vi "IsSetter.vi"(8 "error in (no error)":errorcluster, 10 "Path":path, 11 "ClassReflector in":refnum<class "ClassReflector.lvclass">) -> (0 "error out":errorcluster, 1 "IsSetter?":bool, 3 "ClassReflector out":refnum<class "ClassReflector.lvclass">)   [LabVIEW 2023, in "ClassReflector.lvclass"]
uses:
  ClassReflector.lvclass
  ClassReflector.lvclass/ClassReflector.ctl
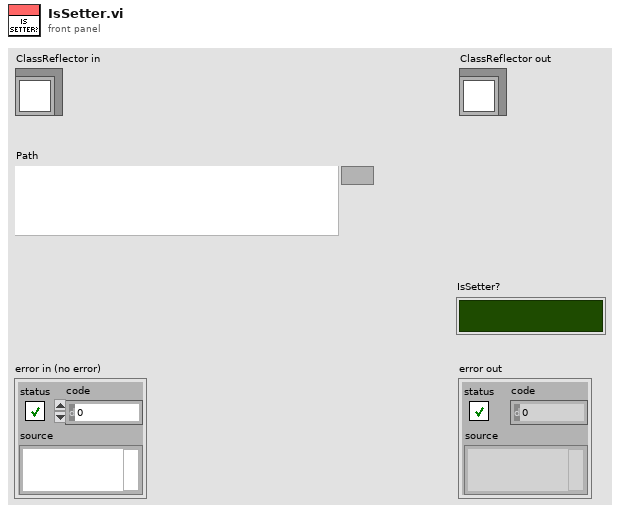
[diagram p1: front panel]
types:
  T1 = enum32{"Bad", "Idle", "Run top level", "Running"}
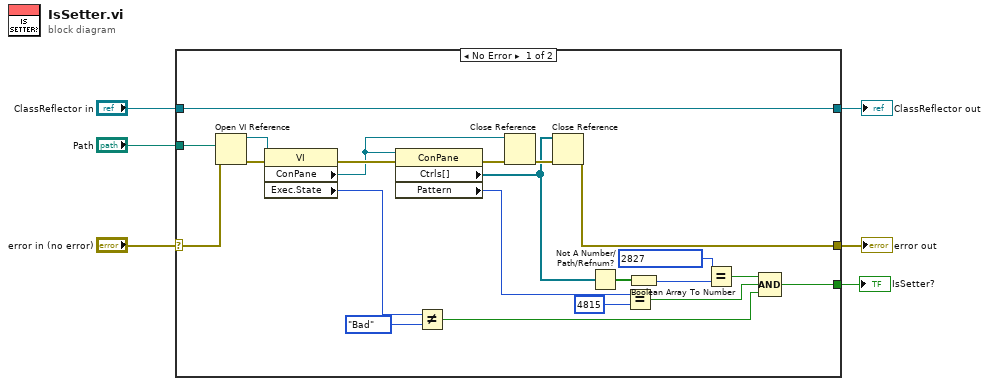
[diagram p0: block diagram]
diagram:
  n1 = case shown="No Error" "error in (no error)" {
    selector: "error in (no error)" -> [w26 w30]
    tunnel: [w7 w30] -> w5
    tunnel: [w28 w29] -> w3
    tunnel: "ClassReflector in" -> [w28 w29]
    tunnel: "Path" -> [w27 _]
    tunnel: [w10 _] -> w1
    frame No Error {
      n2 = Open VI Reference(vi path=w27, error in (no error)=w26) -> (vi reference=w25:refnum<vi>, error out=w24:errorcluster)  [unwired: 4 in]
      n3 = property class="VI"(reference=w25, error in=w24) -> (error out=w23:errorcluster, "ConPane"=w21:refnum<vi>, "Exec.State"=w13:T1)  [unwired: 1 out]
      n4 = property class="ConPane"(reference=w21, error in=w23) -> (error out=w22:errorcluster, "Ctrls[]"=w8:refnum<vi>[], "Pattern"=w20:u32)  [unwired: 1 out]
      n5 = Not Equal?(x=w13, y=T1."Bad") -> (x != y?=w11:bool)
      n6 = Close Reference(reference=w21, error in (no error)=w22) -> (error out=w9:errorcluster)
      n7 = Close Reference(reference=w8, error in (no error)=w9) -> (error out=w7:errorcluster)
      n8 = Not A Number/Path/Refnum?(number/path/refnum=w8) -> (NaN/Path/Refnum?=w19:bool[])
      n9 = Equal?(x=w20, y=u32 4815) -> (x = y?=w14:bool)
      n10 = Boolean Array To Number(Boolean array=w19) -> (number=w18:u32)
      n11 = Equal?(x=u32 2827, y=w18) -> (x = y?=w15:bool)
      n12 = Compound Arithmetic op=AND(w15, w14, w11) -> (w10:bool)
    }
    frame Error {
    }
  }
  "error out" <- w5
  "ClassReflector out" <- w3
  "IsSetter?" <- w1
